vi "HexStringSpaceDelimitAtEveryByte_LV2015.vi"(8 "error in (no error)":errorcluster, 11 "HexString with or without delimitation":string="3qgv5 tsdfg56und 1234 56 7 8 9A BC DEF") -> (0 "error out":errorcluster, 3 "HexByte delimited string":string="35 DF 56 D1 23 45 67 89 AB CD EF")   [LabVIEW 2015]
panel:
  # "Connector Pane"
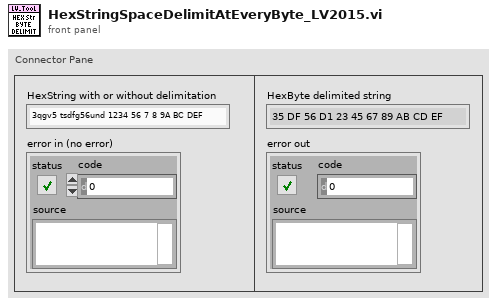
[diagram p1: front panel]
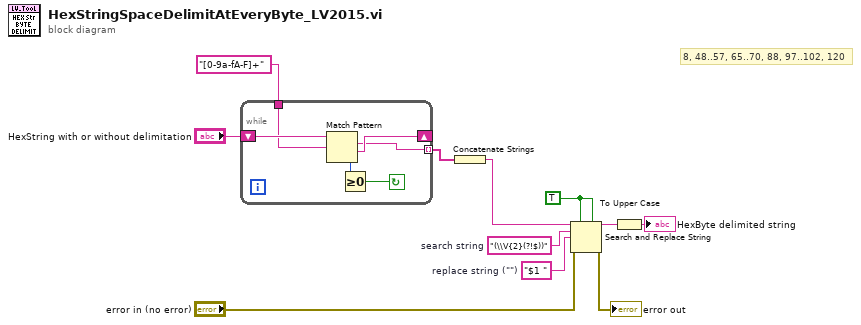
[diagram p0: block diagram]
diagram:
  w8 = TRUE ("replace all? (F)")
  w10 = "$1 "  # replace string ("")
  w11 = "(\\V{2}(?!$))"  # search string
  # "8, 48..57, 65..70, 88, 97..102, 120"
  n1 = while {
    shift-right: [w13] -> _
    shift-left: "HexString with or without delimitation" -> [w17]
    tunnel: "[0-9a-fA-F]+" ("regular expression") -> [w14]
    tunnel: [w12] -> w3 mode=indexing
    stop <- w15 continue-if-true
    n2 = Match Pattern(string=w17, regular expression=w14) -> (match substring=w12:string, after substring=w13:string, offset past match=w16:i32)  [unwired: 2 out]
    n3 = Greater Or Equal To 0?(x=w16) -> (x >= 0?=w15:bool)
  }
  n4 = Concatenate Strings(w3) -> (w2:string)
  n5 = Search and Replace String(replace all?=w8, multiline?=w8, input string=w2, search string=w11, replace string=w10, error in="error in (no error)") -> (result string=w9:string, error out=→"error out":errorcluster)  [unwired: 2 in, 2 out]
  n6 = To Upper Case(1:w9) -> (0:→"HexByte delimited string":string)
